vi "生成波特率.vi"(1 "波特率":i32) -> (0 "GPRS参数":i32 format="%x")   [LabVIEW 2015]
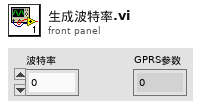
[diagram p1: front panel]
types:
  T1 = typedef "GPRS波特率参数.ctl" = i32[]
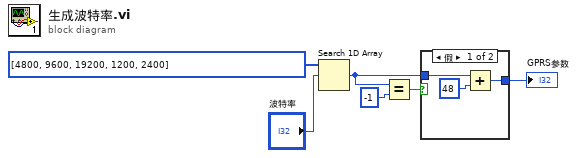
[diagram p0: block diagram]
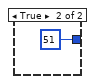
[diagram p2: hidden frame]
diagram:
  n1 = Search 1D Array(1D array=T1 [4800, 9600, 19200, 1200, 2400], element="波特率") -> (index of element=w1:i32)  [unwired: 1 in]
  n2 = Equal?(x=w1, y=-1) -> (x = y?=w3:bool)
  n3 = case shown="假" w3 {
    tunnel: [w8 51] -> w2
    tunnel: w1 -> [w7 _]
    frame False {
      n4 = Add(x=w7, y=u16 48) -> (x+y=w8:i32)
    }
    frame True {
    }
  }
  "GPRS参数" <- w2
